vi "Actor Decorator.vi"(10 "Actor":refnum<class "LVCAM.lvclass">, 11 "Process in":refnum<class "Process.lvclass">) -> (3 "Process out":refnum<class "Process.lvclass">)   [LabVIEW 2021, in "Process.lvlib" / "Process.lvclass"]
uses:
  Process.lvclass
  AAM/AAM/LVCAM/LVCAM.lvclass
  Process.lvclass/Process.ctl
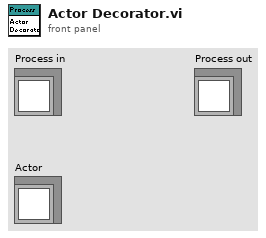
[diagram p1: front panel]
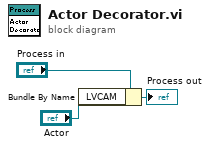
[diagram p0: block diagram]
diagram:
  n1 = Bundle By Name(cluster="Process in", "LVCAM"="Actor") -> (→"Process out":refnum<class "Process.lvclass">)
